vi "auto phase nanonis 2.vi"(0 "Num averages":u32) -> ()   [LabVIEW 2010]
uses:
  <userlib>/Nanonis Prog Interface V5/Nanonis Prog Interface.lvlib
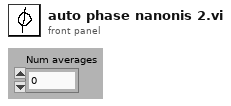
[diagram p1: front panel]
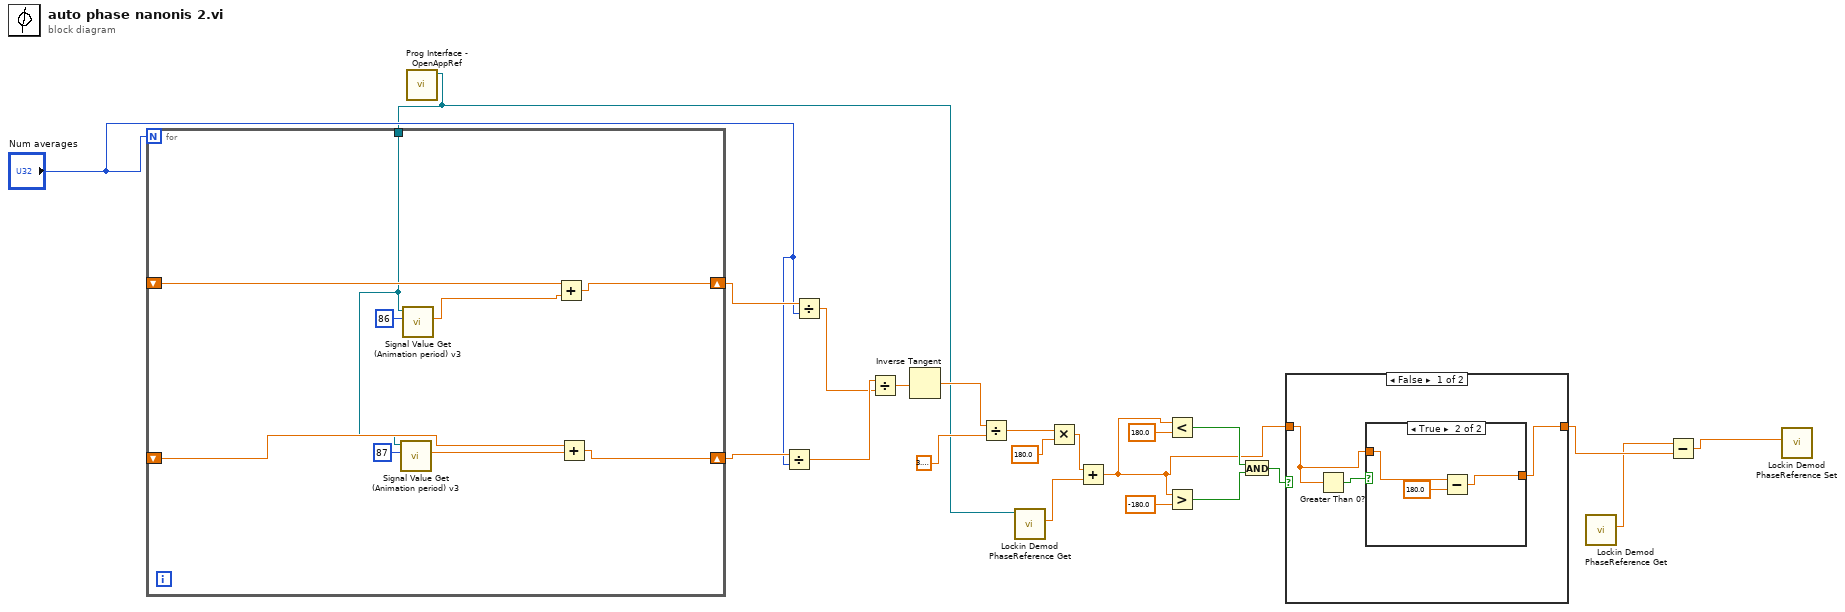
[diagram p0: block diagram]
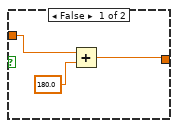
[diagram p2: hidden frame]
diagram:
  n1 = call <userlib>:"Prog Interface - OpenAppRef.vi"() -> ("Application reference"=w10:refnum<vi>)  [unwired: 6 in, 1 out]
  n2 = for {
    N: "Num averages" -> [_]
    shift-right: [w28] -> w22
    shift-left: _ -> [w29]
    shift-right: [w25] -> w21
    shift-left: _ -> [w24]
    tunnel: w10 -> [w23]
    n3 = call <userlib>:"Signal Value Get (Animation period) v3.vi"("Signal index (0-127)"=i8 87, "Application ref in"=w23) -> ("Signal value"=w26:sgl)  [unwired: 6 in, 2 out]
    n4 = call <userlib>:"Signal Value Get (Animation period) v3.vi"("Signal index (0-127)"=i8 86, "Application ref in"=w23) -> ("Signal value"=w30:sgl)  [unwired: 6 in, 2 out]
    n5 = Add(x=w29, y=w30) -> (x+y=w28:sgl)
    n6 = Add(x=w24, y=w26) -> (x+y=w25:sgl)
  }
  n7 = Divide(x=w21, y="Num averages") -> (x/y=w18:sgl)
  n8 = Divide(x=w22, y="Num averages") -> (x/y=w17:sgl)
  n9 = Divide(x=w18, y=w17) -> (x/y=w19:sgl)
  n10 = Inverse Tangent(1:w19) -> (0:w16:sgl)
  n11 = Divide(x=w16, y=3.141592653589793) -> (x/y=w14:dbl)
  n12 = call <userlib>:"Lockin Demod PhaseReference Get.vi"("Application ref in"=w10) -> ("Phase Reference"=w11:sgl)  [unwired: 8 in, 2 out]
  n13 = Multiply(x=w14, y=180.0) -> (x*y=w12:dbl)
  n14 = Add(x=w12, y=w11) -> (x+y=w4:dbl)
  n15 = Less?(x=w4, y=180.0) -> (x < y?=w6:bool)
  n16 = Greater?(x=w4, y=-180.0) -> (0:w7:bool)
  n17 = And(x=w6, y=w7) -> (x .and. y?=w5:bool)
  n18 = case shown="False" w5 {
    tunnel: w4 -> [w33 w41]
    tunnel: [w32 w41] -> w3
    frame False {
      n19 = Greater Than 0?(x=w33) -> (x > 0?=w34:bool)
      n20 = case shown="True" w34 {
        tunnel: w33 -> [w37 w40]
        tunnel: [w35 w38] -> w32
        frame False {
          n21 = Add(x=w37, y=180.0) -> (x+y=w35:dbl)
        }
        frame True {
          n22 = Subtract(x=w40, y=180.0) -> (x-y=w38:dbl)
        }
      }
    }
    frame True {
    }
  }
  n23 = call <userlib>:"Lockin Demod PhaseReference Get.vi"() -> ("Phase Reference"=w2:sgl)  [unwired: 9 in, 2 out]
  n24 = Subtract(x=w2, y=w3) -> (x-y=w1:dbl)
  n25 = call <userlib>:"Lockin Demod PhaseReference Set.vi"("Phase Reference"=w1) -> ()  [unwired: 9 in, 2 out]
